vi "Measurement UI.vi"() -> ()   [LabVIEW 2024, in "Line Regulation_Channel Ganging_UI.lvlib"]
uses:
  Line Regulation_Channel Ganging_UI.lvlib
panel:
  in  "MeasGraphs":T1(tab)
  out "Enabled Sources":string[](array[string])
  out "Enabled Loads":string[](array[string])
  out "LineRegulationGraph(V/V)":T2(graph)
  out "LineRegulationGraph(%)":T3(graph)
  in  "Load current pole-zero ratio":dbl=0.3
  in  "Load current compensation frequency":dbl=180000.0
  in  "Load current gain bandwidth":dbl=14000.0
  in  "Source voltage pole-zero ratio":dbl=2.0
  in  "Source voltage compensation frequency":dbl=3530.0
  in  "Source voltage gain bandwidth":dbl=2000.0
  out "Load voltage deviation":dbl[](array[numeric])
  out "Ganged load voltages":dbl[](array[numeric])
  out "Ganged source voltages":dbl[](array[numeric])
  in  "Load slave resource names":string[](array[string])
  in  "Load master resource name":string
  in  "Source slave resource names":string[](array[string])
  in  "Source master resource name":string
  in  "Mode of operation":T4(ring)=enum."Perform measurement" caption="MODE OF OPERATION"
  in  "MeasConfigurations":T5(tab)=enum."Source Config"
  in  "Measurement timeout":dbl=10.0 caption="MEASUREMENT TIMEOUT" format="%.3ps"
  in  "Nominal output voltage":dbl=1.0 caption="NOMINAL OUTPUT VOLTAGE" format="%.3pV"
  in  "Source delay":dbl=0.005 caption="SOURCE DELAY" format="%.3ps"
  in  "DUT setup time":dbl=1.0 caption="DUT SETUP TIME" format="%.3ps"
  in  "Aperture time":dbl=0.005 caption="APERTURE TIME" format="%.3ps"
  in  "PPSSlaveResourceNames":refnum<k15>[](array[refnum]) caption="SLAVE RESOURCE NAMES"
  in  "PPSMasterResourceName":refnum<k15> caption="MASTER RESOURCE NAME"
  in  "Source stop voltage":dbl=14.0 caption="VOLTAGE STOP LEVEL" format="%#_6pV"
  in  "Source transient response":i32(ring)=1038 caption="TRANSIENT RESPONSE" items=["Slow"=1041, "Normal"=1038, "Fast"=1039, "Custom"=1042]
  in  "Source sense":i32(ring)=1009 caption="SENSE" items=["Local"=1008, "Remote"=1009]
  in  "Source voltage level range":dbl=20.0 caption="VOLTAGE LEVEL RANGE" format="%#_6pV"
  in  "Source start voltage":dbl=6.0 caption="VOLTAGE START LEVEL" format="%#_6pV"
  in  "Source current limit high":dbl=25.0 caption="CURRENT LIMIT/LIMIT HIGH" format="%#_6pA"
  in  "Source current limit range":dbl=25.0 caption="CURRENT LIMIT RANGE" format="%#_6pA"
  in  "Source limit symmetry":enum32{"Symmetric", "Asymmetric"}(ring)=enum."Asymmetric" caption="LIMIT SYMMETRY"
  in  "Source current limit low":dbl=-0.6 caption="CURRENT LIMIT LOW" format="%#_6pA"
  in  "Source system configuration":enum32{"Series", "Parallel"}(ring)=enum."Parallel" caption="SYSTEM CONFIG"
  in  "Source compliance":string="Compliance"
  in  "Source sourceadapt":string="SourceAdapt"
  in  "Source Custom Transient Response":bool
  in  "Source sweep type":string(combo)="Logarithmic" caption="SWEEP TYPE"
  in  "Source current sweep points/points per decade":i32=10 caption="PTS/PTS PER DECADE"
  out "Status":string
  in  "Load current level":dbl=1.0 caption="CURRENT LEVEL" format="%#_6pA"
  in  "Load sourceadapt":string="SourceAdapt"
  in  "Load compliance":string="Compliance"
  in  "Load system configuration":enum32{"Series", "Parallel"}(ring)=enum."Parallel" caption="SYSTEM CONFIG"
  in  "Load voltage limit low":dbl caption="VOLTAGE  LIMIT LOW" format="%#_6pV"
  in  "Load limit symmetry":enum32{"Symmetric", "Asymmetric"}(ring) caption="LIMIT SYMMETRY"
  in  "Load voltage limit range":dbl=6.0 caption="VOLTAGE LIMIT RANGE" format="%#_6pV"
  in  "Load voltage limit high":dbl=inf caption="VOLTAGE LIMIT/LIMIT HIGH" format="%#_6p"
  in  "Load current level range":dbl=80.0 caption="CURRENT LEVEL RANGE" format="%#_6pA"
  in  "Load sense":i32(ring)=1009 caption="SENSE" items=["Local"=1008, "Remote"=1009]
  in  "Load transient response":i32(ring)=1038 caption="TRANSIENT RESPONSE" items=["Slow"=1041, "Normal"=1038, "Fast"=1039, "Custom"=1042]
  in  "LoadSlaveResourceNames":refnum<k15>[](array[refnum]) caption="SLAVE RESOURCE NAMES"
  in  "LoadMasterResourceName":refnum<k15> caption="MASTER RESOURCE NAME"
  in  "Load Custom Transient Response":bool
  out "Status (Load)":string
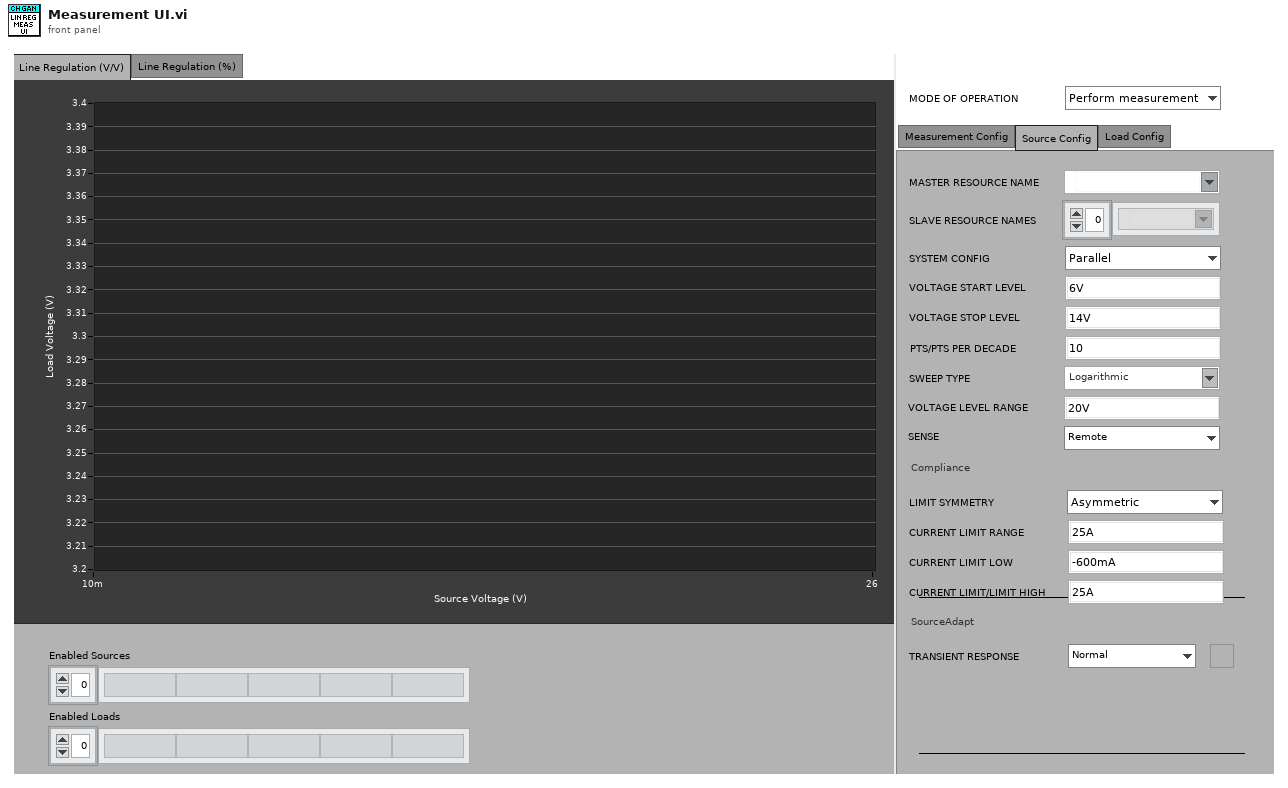
[diagram p1: front panel]
types:
  T1 = enum32{"Line Regulation (V/V)", "Line Regulation (%)", "Hidden Controls"}
  T2 = cluster{"Source voltages":dbl[], "Load voltages":dbl[]}
  T3 = cluster{"Source voltages":dbl[], "Load voltage deviation":dbl[]}
  T4 = enum32{"Power on the DUT", "Perform measurement", "Power off the DUT"}
  T5 = enum32{"Measurement Config", "Source Config", "Load Config"}
  T6 = typedef "SourceAdapt Parameters.ctl" = cluster{"Voltage gain bandwidth":dbl, "Voltage compensation frequency":dbl, "Voltage pole-zero ratio":dbl, "Current gain bandwidth":dbl, "Current compensation frequency":dbl, "Current pole-zero ratio":dbl}
  T7 = cluster{"Ganged source voltages":dbl[], "Ganged load voltages":dbl[]}
  T8 = cluster{"Ganged source voltages":dbl[], "Load voltage deviation":dbl[]}
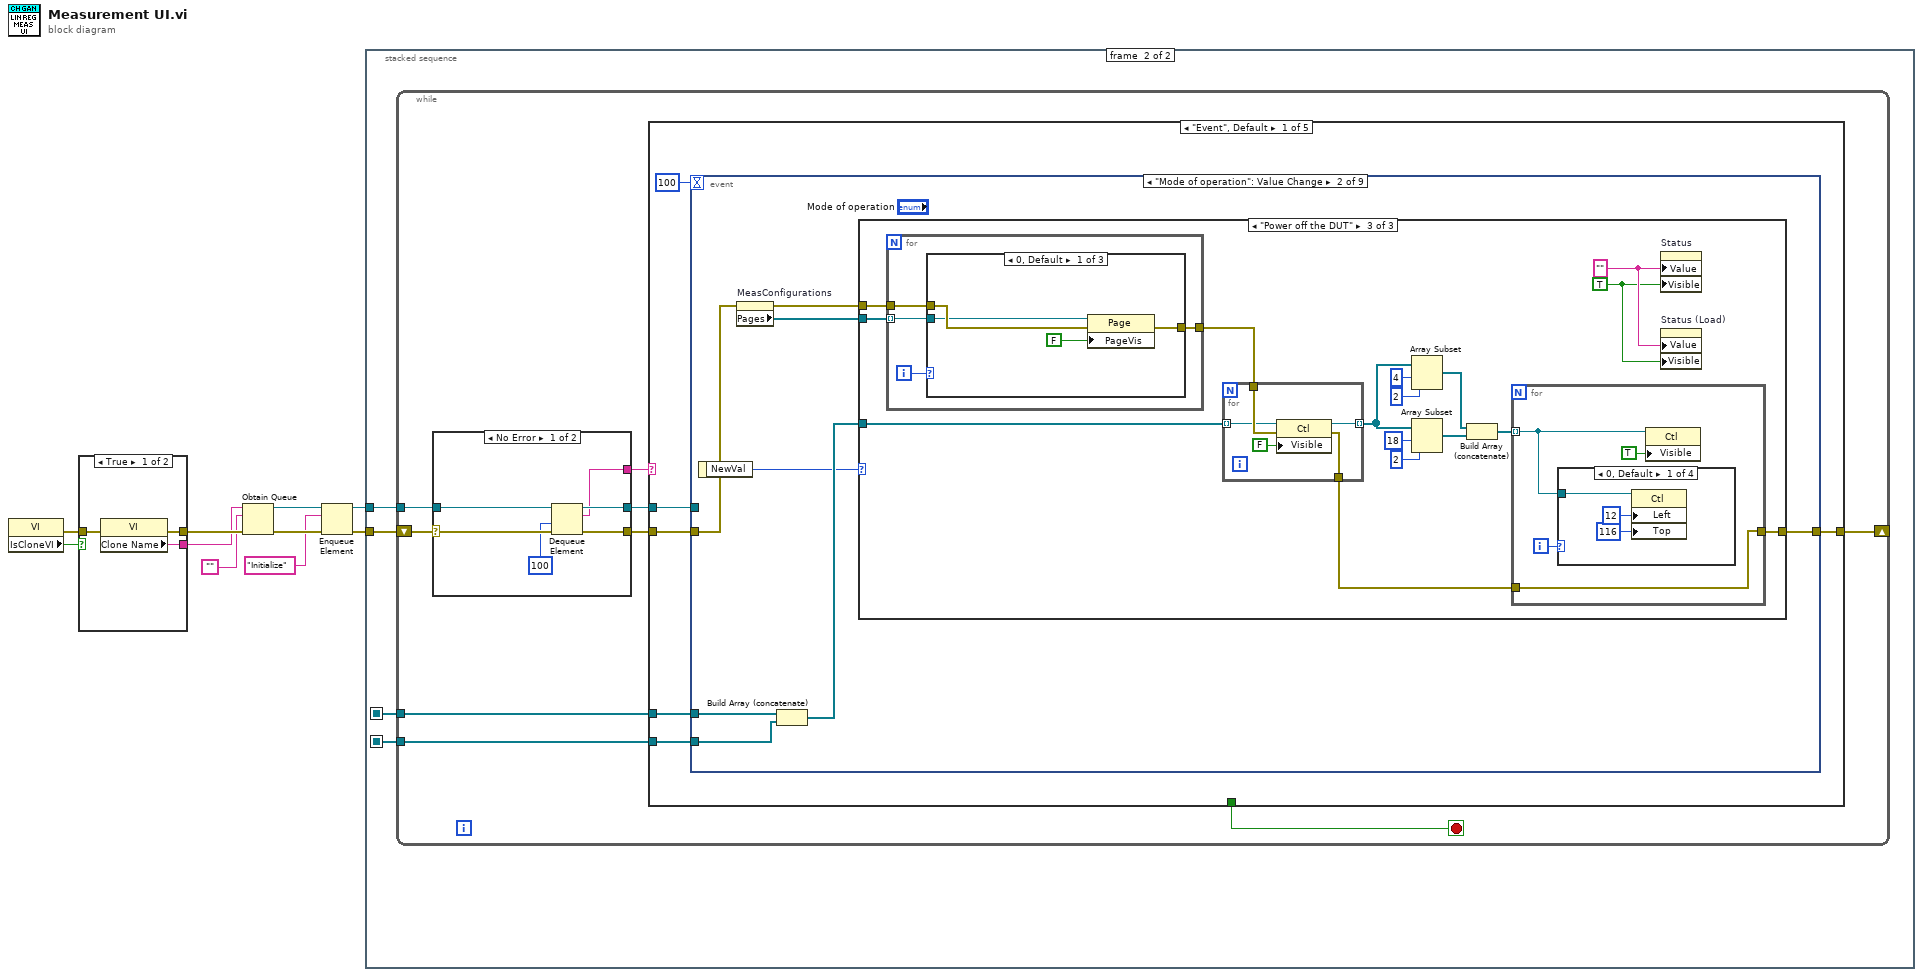
[diagram p0: block diagram]
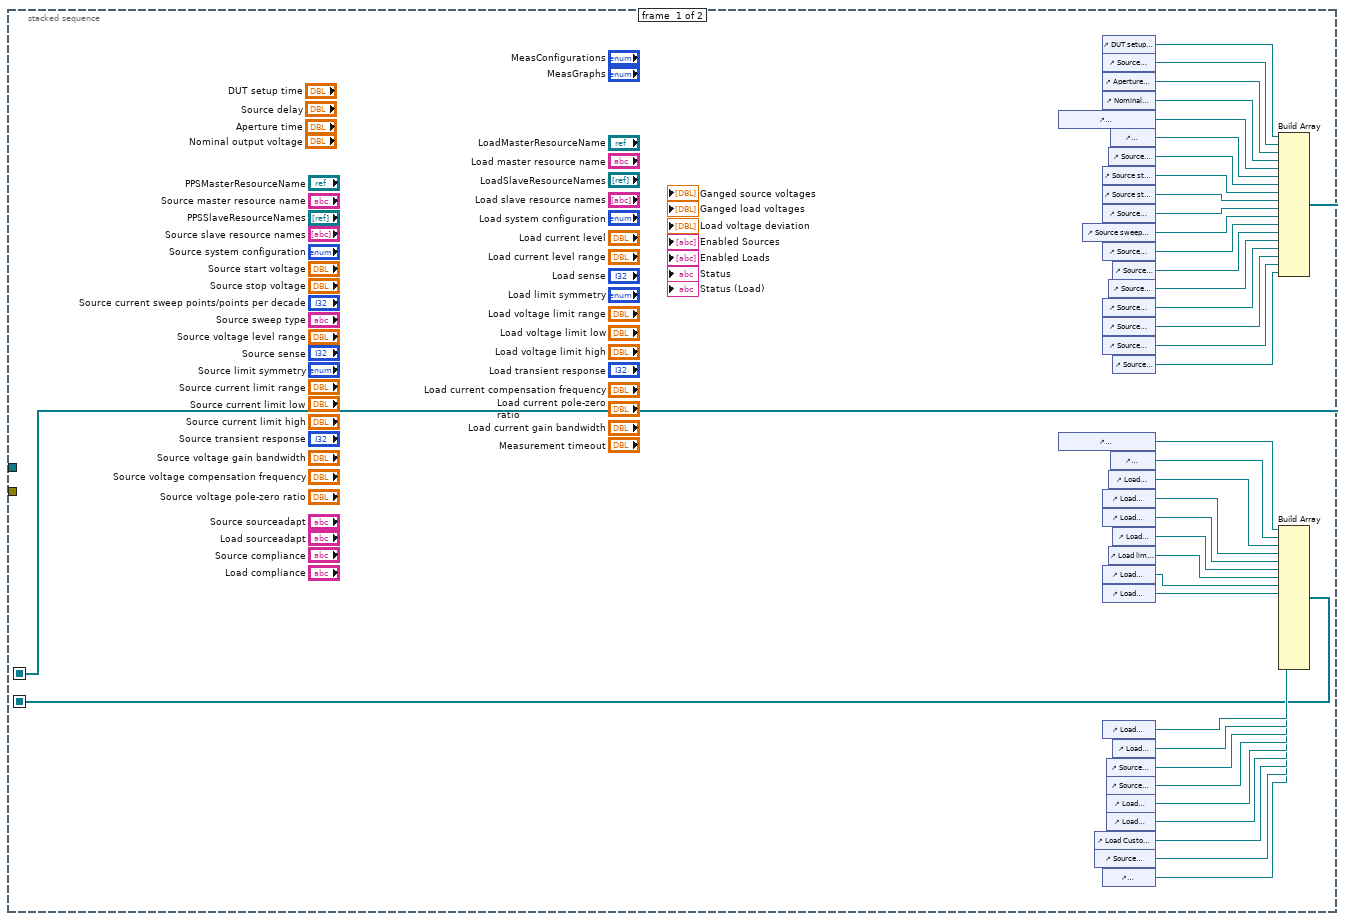
[diagram p2: hidden frame]
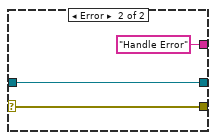
[diagram p3: hidden frame]
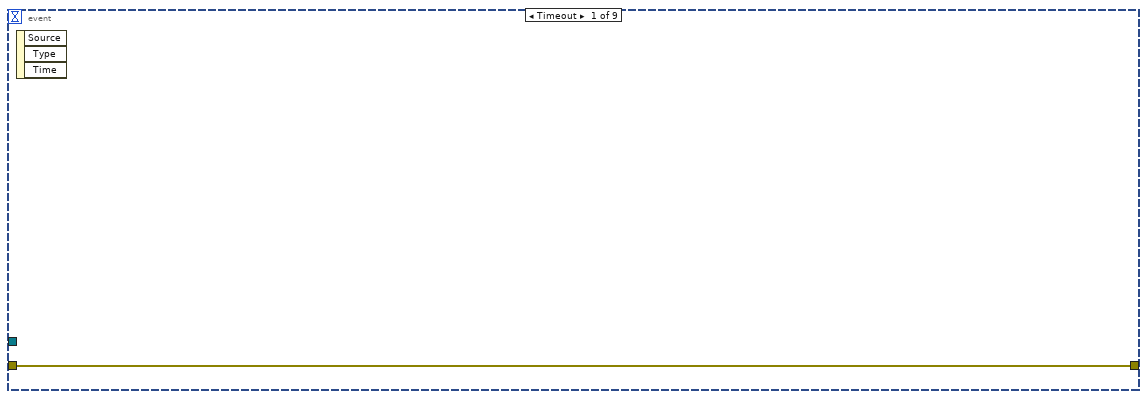
[diagram p4: hidden frame]
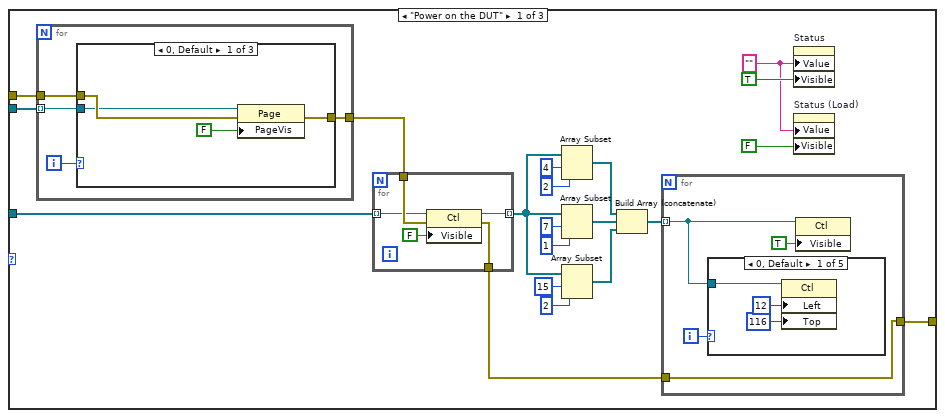
[diagram p5: hidden frame]
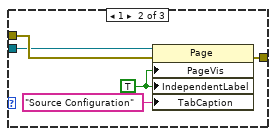
[diagram p6: hidden frame]
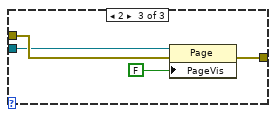
[diagram p7: hidden frame]
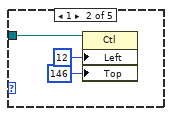
[diagram p8: hidden frame]
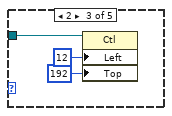
[diagram p9: hidden frame]
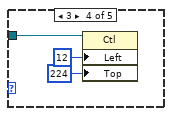
[diagram p10: hidden frame]
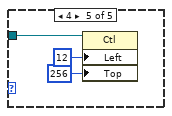
[diagram p11: hidden frame]
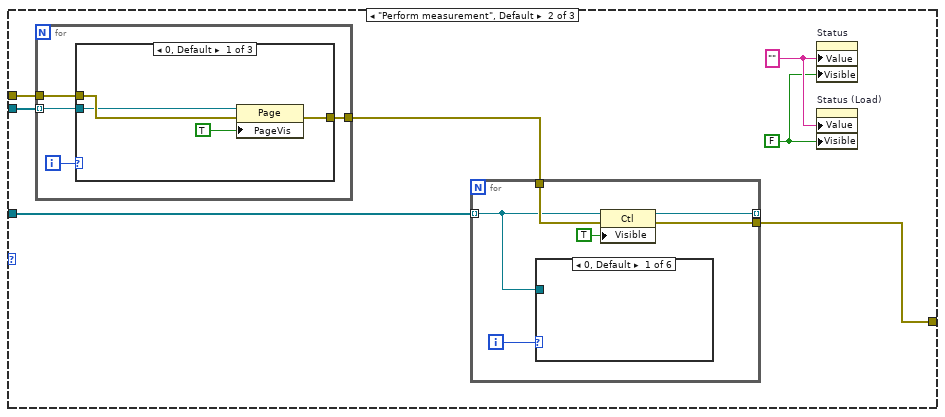
[diagram p12: hidden frame]
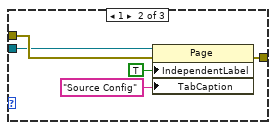
[diagram p13: hidden frame]
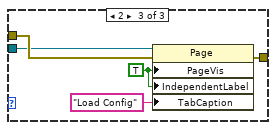
[diagram p14: hidden frame]
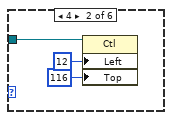
[diagram p15: hidden frame]
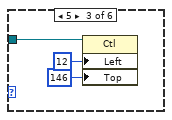
[diagram p16: hidden frame]
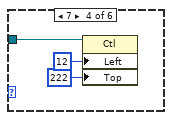
[diagram p17: hidden frame]
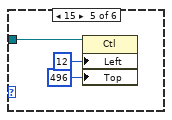
[diagram p18: hidden frame]
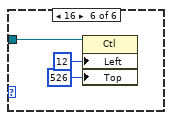
[diagram p19: hidden frame]
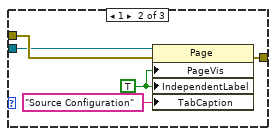
[diagram p20: hidden frame]
diagram:
  n1 = property class="VI"() -> (error out=w1:errorcluster, "IsCloneVI"=w2:bool)  [unwired: 2 in, 1 out]
  n2 = case shown="True" w2 {
    tunnel: [w13 w16] -> w10
    tunnel: [w12 w15] -> w9
    tunnel: w1 -> [w11 w14]
    frame True {
      n3 = property class="VI"(error in=w11) -> (error out=w13:errorcluster, "Clone Name"=w12:string)  [unwired: 1 in, 1 out]
    }
    frame False {
      n4 = property class="VI"(error in=w14) -> (error out=w16:errorcluster, "Name"=w15:string)  [unwired: 1 in, 1 out]
    }
  }
  n5 = Obtain Queue(name (unnamed)=w9, element data type="", error in (no error)=w10) -> (queue out=w6:refnum<queue>, error out=w8:errorcluster)  [unwired: 2 in, 1 out]
  n6 = Enqueue Element(queue=w6, element="Initialize", error in (no error)=w8) -> (queue out=w5:refnum<queue>, error out=w7:errorcluster)  [unwired: 1 in, 1 out]
  n7 = stacked-sequence {
    seq-local: [w18 _] -> [_ w56]
    seq-local: [w17 _] -> [_ w55]
    tunnel: w7 -> [_ w58]
    tunnel: w5 -> [_ w57]
    frame #0 {
      n8 = control-ref of="PPSMasterResourceName"() -> (w50:refnum<vi>)
      n9 = control-ref of="LoadMasterResourceName"() -> (w36:refnum<vi>)
      n10 = control-ref of="Source sweep type"() -> (w44:refnum<vi>)
      n11 = control-ref of="Load Custom Transient Response"() -> (w21:refnum<vi>)
      n12 = control-ref of="Source Custom Transient Response"() -> (w20:refnum<vi>)
      n13 = control-ref of="DUT setup time"() -> (w54:refnum<vi>)
      n14 = control-ref of="Source delay"() -> (w53:refnum<vi>)
      n15 = control-ref of="Aperture time"() -> (w52:refnum<vi>)
      n16 = control-ref of="Nominal output voltage"() -> (w51:refnum<vi>)
      n17 = control-ref of="Source start voltage"() -> (w47:refnum<vi>)
      n18 = control-ref of="Source stop voltage"() -> (w46:refnum<vi>)
      n19 = control-ref of="Source current sweep points/points per decade"() -> (w45:refnum<vi>)
      n20 = control-ref of="Source voltage level range"() -> (w43:refnum<vi>)
      n21 = control-ref of="Source current limit range"() -> (w40:refnum<vi>)
      n22 = control-ref of="Source current limit low"() -> (w39:refnum<vi>)
      n23 = control-ref of="Source current limit high"() -> (w38:refnum<vi>)
      n24 = control-ref of="Load current level"() -> (w33:refnum<vi>)
      n25 = control-ref of="Load current level range"() -> (w32:refnum<vi>)
      n26 = control-ref of="Load voltage limit range"() -> (w29:refnum<vi>)
      n27 = control-ref of="Load voltage limit low"() -> (w28:refnum<vi>)
      n28 = control-ref of="Load voltage limit high"() -> (w27:refnum<vi>)
      n29 = control-ref of="Measurement timeout"() -> (w19:refnum<vi>)
      n30 = control-ref of="Source compliance"() -> (w25:refnum<vi>)
      n31 = control-ref of="Source sourceadapt"() -> (w24:refnum<vi>)
      n32 = control-ref of="Load compliance"() -> (w23:refnum<vi>)
      n33 = control-ref of="Load sourceadapt"() -> (w22:refnum<vi>)
      n34 = control-ref of="Source system configuration"() -> (w48:refnum<vi>)
      n35 = control-ref of="Source limit symmetry"() -> (w41:refnum<vi>)
      n36 = control-ref of="Load system configuration"() -> (w34:refnum<vi>)
      n37 = control-ref of="Load limit symmetry"() -> (w30:refnum<vi>)
      n38 = control-ref of="PPSSlaveResourceNames"() -> (w49:refnum<vi>)
      n39 = control-ref of="LoadSlaveResourceNames"() -> (w35:refnum<vi>)
      n40 = control-ref of="Source sense"() -> (w42:refnum<vi>)
      n41 = control-ref of="Source transient response"() -> (w37:refnum<vi>)
      n42 = control-ref of="Load sense"() -> (w31:refnum<vi>)
      n43 = control-ref of="Load transient response"() -> (w26:refnum<vi>)
      n44 = Build Array(w54, w53, w52, w51, w50, w49, w48, w47, w46, w45, w44, w43, w42, w41, w40, w39, w38, w37) -> (w18:refnum<vi>[])
      n45 = Build Array(w36, w35, w34, w33, w32, w31, w30, w29, w28, w27, w26, w25, w24, w23, w22, w21, w20, w19) -> (w17:refnum<vi>[])
    }
    frame #1 {
      n46 = while {
        shift-right: [w62] -> _
        shift-left: w58 -> [w67]
        tunnel: w57 -> [w65]
        tunnel: w56 -> [w60]
        tunnel: w55 -> [w59]
        stop <- w61 stop-if-true
        n47 = case shown="No Error" w67 {
          selector: w67 -> [w73 w76]
          tunnel: [w72 w76] -> w66
          tunnel: w65 -> [w71 w75]
          tunnel: [w70 w75] -> w64
          tunnel: [w69 "Handle Error"] -> w63
          frame No Error {
            n48 = Dequeue Element(queue=w71, timeout in ms (-1)=100, error in (no error)=w73) -> (queue out=w70:refnum<queue>, element=w69:string, error out=w72:errorcluster)  [unwired: 1 out]
          }
          frame Error {
          }
        }
        n49 = case shown="\"Event\", Default" w63 {
          tunnel: w66 -> [w81 w272 w285 w294 w295]
          tunnel: w64 -> [w79 _ _ w292 _]
          tunnel: [w82 w272 w285 w289 w295] -> w62
          tunnel: [_ FALSE _ TRUE _] -> w61
          tunnel: w60 -> [w78 _ _ _ _]
          tunnel: w59 -> [w77 _ _ _ _]
          frame "Event", Default {
            n50 = event shown="[1] \"Mode of operation\": Value Change" {
              selector: _ -> [_ _ _ _ _ _ _ _ _]
              dyn-events: _ -> [_ _ _ _ _ _ _ _ _]
              timeout: 100 -> [_ _ _ _ _ _ _ _ _]
              tunnel: [w83 w90 _ _ _ _ _ _ w268] -> w82
              tunnel: w81 -> [w83 w84 _ _ _ _ _ _ w269]
              tunnel: w79 -> [_ _ _ _ _ _ _ _ w267]
              tunnel: w78 -> [_ w88 _ _ _ _ _ _ _]
              tunnel: w77 -> [_ w87 _ _ _ _ _ _ _]
              event Timeout {
                n51 = event-data() -> ()  [unwired: 1 in, 3 out]
              }
              event "Mode of operation": Value Change {
                n52 = event-data() -> ("NewVal"=w89:T4)  [unwired: 1 in]
                n53 = property on="MeasConfigurations" class="TabCtl (strict)"(error in=w84) -> (error out=w85:errorcluster, "Pages"=w86:refnum<vi>[])  [unwired: 1 in, 1 out]
                n54 = Build Array (concatenate)(w88, w87) -> (w91:refnum<vi>[])
                n55 = case shown="\"Power off the DUT\"" w89 {
                  tunnel: w91 -> [w111 w159 w214]
                  tunnel: w86 -> [w99 w158 w209]
                  tunnel: w85 -> [w98 w157 w208]
                  tunnel: [w95 w155 w205] -> w90
                  frame "Power on the DUT" {
                    w93 = ""
                    n56 = for {
                      tunnel: w99 -> [w114] mode=indexing
                      tunnel: w98 -> [w113]
                      tunnel: [w112] -> w97
                      i -> [w115]
                      n57 = case shown="0, Default" w115 {
                        tunnel: w114 -> [w118 w123 w127]
                        tunnel: w113 -> [w119 w124 w128]
                        tunnel: [w116 w121 w125] -> w112
                        frame 0, Default {
                          n58 = property class="Page"(reference=w118, error in=w119, "PageVis"=FALSE ("Independent Label")) -> (error out=w116:errorcluster)  [unwired: 1 out]
                        }
                        frame 1 {
                          w120 = TRUE ("Independent Label")
                          n59 = property class="Page"(reference=w123, error in=w124, "PageVis"=w120, "IndependentLabel"=w120, "TabCaption"="Source Configuration" ("Tab Caption")) -> (error out=w121:errorcluster)  [unwired: 1 out]
                        }
                        frame 2 {
                          n60 = property class="Page"(reference=w127, error in=w128, "PageVis"=FALSE ("Independent Label")) -> (error out=w125:errorcluster)  [unwired: 1 out]
                        }
                      }
                    }
                    n61 = for {
                      tunnel: w111 -> [w151] mode=indexing
                      tunnel: [w149] -> w104 mode=indexing
                      tunnel: w97 -> [w152]
                      tunnel: [w148] -> w96
                      n62 = property class="Ctl"(reference=w151, error in=w152, "Visible"=FALSE) -> (reference out=w149:refnum<vi>, error out=w148:errorcluster)
                    }
                    n63 = Array Subset(array=w104, index=4, length=2) -> (w102:refnum<vi>[])
                    n64 = Array Subset(array=w104, index=7, length=1) -> (w103:refnum<vi>[])
                    n65 = Array Subset(array=w104, index=15, length=2) -> (w101:refnum<vi>[])
                    n66 = Build Array (concatenate)(w102, w103, w101) -> (w100:refnum<vi>[])
                    n67 = for {
                      tunnel: w100 -> [w130] mode=indexing
                      tunnel: w96 -> [w129]
                      tunnel: [w129] -> w95
                      i -> [w131]
                      n68 = case shown="0, Default" w131 {
                        tunnel: w130 -> [w135 w138 w141 w144 w147]
                        frame 0, Default {
                          n69 = property class="Ctl"(reference=w135, "Left"=12 ("Position:Left"), "Top"=116 ("Position:Left")) -> ()  [unwired: 1 in, 2 out]
                        }
                        frame 1 {
                          n70 = property class="Ctl"(reference=w138, "Left"=12 ("Position:Left"), "Top"=146 ("Position:Left")) -> ()  [unwired: 1 in, 2 out]
                        }
                        frame 2 {
                          n71 = property class="Ctl"(reference=w141, "Left"=12 ("Position:Left"), "Top"=192 ("Position:Left")) -> ()  [unwired: 1 in, 2 out]
                        }
                        frame 3 {
                          n72 = property class="Ctl"(reference=w144, "Left"=12 ("Position:Left"), "Top"=224 ("Position:Left")) -> ()  [unwired: 1 in, 2 out]
                        }
                        frame 4 {
                          n73 = property class="Ctl"(reference=w147, "Left"=12 ("Position:Left"), "Top"=256 ("Position:Left")) -> ()  [unwired: 1 in, 2 out]
                        }
                      }
                      n74 = property class="Ctl"(reference=w130, "Visible"=TRUE) -> ()  [unwired: 1 in, 2 out]
                    }
                    n75 = property on="Status" class="Str"("Value"=w93, "Visible"=TRUE) -> ()  [unwired: 2 in, 2 out]
                    n76 = property on="Status (Load)" class="Str"("Value"=w93, "Visible"=FALSE) -> ()  [unwired: 2 in, 2 out]
                  }
                  frame "Perform measurement", Default {
                    w153 = FALSE ("Visible")
                    w154 = ""
                    n77 = for {
                      tunnel: w158 -> [w162] mode=indexing
                      tunnel: w157 -> [w161]
                      tunnel: [w160] -> w156
                      i -> [w163]
                      n78 = case shown="0, Default" w163 {
                        tunnel: w162 -> [w166 w171 w176]
                        tunnel: w161 -> [w167 w172 w177]
                        tunnel: [w164 w168 w175] -> w160
                        frame 0, Default {
                          n79 = property class="Page"(reference=w166, error in=w167, "PageVis"=TRUE ("Independent Label")) -> (error out=w164:errorcluster)  [unwired: 1 out]
                        }
                        frame 1 {
                          n80 = property class="Page"(reference=w171, error in=w172, "IndependentLabel"=TRUE ("Independent Label"), "TabCaption"="Source Config" ("Tab Caption")) -> (error out=w168:errorcluster)  [unwired: 1 out]
                        }
                        frame 2 {
                          w174 = TRUE ("Independent Label")
                          n81 = property class="Page"(reference=w176, error in=w177, "PageVis"=w174, "IndependentLabel"=w174, "TabCaption"="Load Config" ("Tab Caption")) -> (error out=w175:errorcluster)  [unwired: 1 out]
                        }
                      }
                    }
                    n82 = for {
                      tunnel: w159 -> [w179] mode=indexing
                      tunnel: [w181] -> _ mode=indexing
                      tunnel: w156 -> [w183]
                      tunnel: [w178] -> w155
                      i -> [w180]
                      n83 = case shown="0, Default" w180 {
                        tunnel: w179 -> [_ w186 w189 w192 w195 w198]
                        frame 0, Default {
                        }
                        frame 4 {
                          n84 = property class="Ctl"(reference=w186, "Left"=12 ("Position:Left"), "Top"=116 ("Position:Left")) -> ()  [unwired: 1 in, 2 out]
                        }
                        frame 5 {
                          n85 = property class="Ctl"(reference=w189, "Left"=12 ("Position:Left"), "Top"=146 ("Position:Left")) -> ()  [unwired: 1 in, 2 out]
                        }
                        frame 7 {
                          n86 = property class="Ctl"(reference=w192, "Left"=12 ("Position:Left"), "Top"=222 ("Position:Left")) -> ()  [unwired: 1 in, 2 out]
                        }
                        frame 15 {
                          n87 = property class="Ctl"(reference=w195, "Left"=12 ("Position:Left"), "Top"=496 ("Position:Left")) -> ()  [unwired: 1 in, 2 out]
                        }
                        frame 16 {
                          n88 = property class="Ctl"(reference=w198, "Left"=12 ("Position:Left"), "Top"=526 ("Position:Left")) -> ()  [unwired: 1 in, 2 out]
                        }
                      }
                      n89 = property class="Ctl"(reference=w179, error in=w183, "Visible"=TRUE) -> (reference out=w181:refnum<vi>, error out=w178:errorcluster)
                    }
                    n90 = property on="Status" class="Str"("Value"=w154, "Visible"=w153) -> ()  [unwired: 2 in, 2 out]
                    n91 = property on="Status (Load)" class="Str"("Value"=w154, "Visible"=w153) -> ()  [unwired: 2 in, 2 out]
                  }
                  frame "Power off the DUT" {
                    w199 = TRUE
                    w200 = ""
                    n92 = for {
                      tunnel: w209 -> [w217] mode=indexing
                      tunnel: w208 -> [w216]
                      tunnel: [w215] -> w207
                      i -> [w218]
                      n93 = case shown="0, Default" w218 {
                        tunnel: w217 -> [w221 w226 w231]
                        tunnel: w216 -> [w222 w227 w232]
                        tunnel: [w219 w224 w229] -> w215
                        frame 0, Default {
                          n94 = property class="Page"(reference=w221, error in=w222, "PageVis"=FALSE ("Independent Label")) -> (error out=w219:errorcluster)  [unwired: 1 out]
                        }
                        frame 1 {
                          w223 = TRUE ("Independent Label")
                          n95 = property class="Page"(reference=w226, error in=w227, "PageVis"=w223, "IndependentLabel"=w223, "TabCaption"="Source Configuration" ("Tab Caption")) -> (error out=w224:errorcluster)  [unwired: 1 out]
                        }
                        frame 2 {
                          w228 = TRUE ("Independent Label")
                          n96 = property class="Page"(reference=w231, error in=w232, "PageVis"=w228, "IndependentLabel"=w228, "TabCaption"="Load Configuration" ("Tab Caption")) -> (error out=w229:errorcluster)  [unwired: 1 out]
                        }
                      }
                    }
                    n97 = for {
                      tunnel: w214 -> [w252] mode=indexing
                      tunnel: [w250] -> w202 mode=indexing
                      tunnel: w207 -> [w253]
                      tunnel: [w249] -> w206
                      n98 = property class="Ctl"(reference=w252, error in=w253, "Visible"=FALSE) -> (reference out=w250:refnum<vi>, error out=w249:errorcluster)
                    }
                    n99 = Array Subset(array=w202, index=4, length=2) -> (w211:refnum<vi>[])
                    n100 = Array Subset(array=w202, index=18, length=2) -> (w201:refnum<vi>[])
                    n101 = Build Array (concatenate)(w211, w201) -> (w210:refnum<vi>[])
                    n102 = for {
                      tunnel: w210 -> [w234] mode=indexing
                      tunnel: w206 -> [w233]
                      tunnel: [w233] -> w205
                      i -> [w235]
                      n103 = case shown="0, Default" w235 {
                        tunnel: w234 -> [w239 w242 w245 w248]
                        frame 0, Default {
                          n104 = property class="Ctl"(reference=w239, "Left"=12 ("Position:Left"), "Top"=116 ("Position:Left")) -> ()  [unwired: 1 in, 2 out]
                        }
                        frame 1 {
                          n105 = property class="Ctl"(reference=w242, "Left"=12 ("Position:Left"), "Top"=146 ("Position:Left")) -> ()  [unwired: 1 in, 2 out]
                        }
                        frame 2 {
                          n106 = property class="Ctl"(reference=w245, "Left"=12 ("Position:Left"), "Top"=116 ("Position:Left")) -> ()  [unwired: 1 in, 2 out]
                        }
                        frame 3 {
                          n107 = property class="Ctl"(reference=w248, "Left"=12 ("Position:Left"), "Top"=146 ("Position:Left")) -> ()  [unwired: 1 in, 2 out]
                        }
                      }
                      n108 = property class="Ctl"(reference=w234, "Visible"=TRUE) -> ()  [unwired: 1 in, 2 out]
                    }
                    n109 = property on="Status" class="Str"("Value"=w200, "Visible"=w199) -> ()  [unwired: 2 in, 2 out]
                    n110 = property on="Status (Load)" class="Str"("Value"=w200, "Visible"=w199) -> ()  [unwired: 2 in, 2 out]
                  }
                }
              }
              event "PPSMasterResourceName": Value Change {
                n111 = event-data() -> ("NewVal"=w254:refnum<k15>)  [unwired: 1 in]
                n112 = property on="Source master resource name" class="Str"("Value"=w254) -> ()  [unwired: 2 in, 2 out]
              }
              event "PPSSlaveResourceNames": Value Change {
                n113 = event-data() -> ("NewVal"=w255:refnum<k15>[])  [unwired: 1 in]
                n114 = property on="Source slave resource names" class="Arr (strict)"("Value"=w255) -> ()  [unwired: 2 in, 2 out]
              }
              event "LoadMasterResourceName": Value Change {
                n115 = event-data() -> ("NewVal"=w256:refnum<k15>)  [unwired: 1 in]
                n116 = property on="Load master resource name" class="Str"("Value"=w256) -> ()  [unwired: 2 in, 2 out]
              }
              event "LoadSlaveResourceNames": Value Change {
                n117 = event-data() -> ("NewVal"=w257:refnum<k15>[])  [unwired: 1 in]
                n118 = property on="Load slave resource names" class="Arr (strict)"("Value"=w257) -> ()  [unwired: 2 in, 2 out]
              }
              event "Source Custom Transient Response": Value Change {
                n119 = event-data() -> ()  [unwired: 1 in, 6 out]
                n120 = call "Custom Transient Response for Sweep & Single Point.vi"() -> ("SourceAdapt Parameters"=w261:T6)  [unwired: 11 in]
                n121 = Unbundle By Name(w261) -> ("Voltage gain bandwidth"=w260:dbl, "Voltage compensation frequency"=w259:dbl, "Voltage pole-zero ratio"=w258:dbl)
                n122 = property on="Source voltage gain bandwidth" class="DigNum (strict)"("Value"=w260) -> ()  [unwired: 2 in, 2 out]
                n123 = property on="Source voltage compensation frequency" class="DigNum (strict)"("Value"=w259) -> ()  [unwired: 2 in, 2 out]
                n124 = property on="Source voltage pole-zero ratio" class="DigNum (strict)"("Value"=w258) -> ()  [unwired: 2 in, 2 out]
              }
              event "Load Custom Transient Response": Value Change {
                n125 = event-data() -> ()  [unwired: 1 in, 6 out]
                n126 = call "Custom Transient Response for Sweep & Single Point.vi"() -> ("SourceAdapt Parameters"=w265:T6)  [unwired: 11 in]
                n127 = Unbundle By Name(w265) -> ("Current gain bandwidth"=w264:dbl, "Current compensation frequency"=w263:dbl, "Current pole-zero ratio"=w262:dbl)
                n128 = property on="Load current gain bandwidth" class="DigNum (strict)"("Value"=w264) -> ()  [unwired: 2 in, 2 out]
                n129 = property on="Load current compensation frequency" class="DigNum (strict)"("Value"=w263) -> ()  [unwired: 2 in, 2 out]
                n130 = property on="Load current pole-zero ratio" class="DigNum (strict)"("Value"=w262) -> ()  [unwired: 2 in, 2 out]
              }
              event Panel Close? {
                n131 = event-data() -> ()  [unwired: 1 in, 4 out]
                n132 = Enqueue Element(queue=w267, element="Exit", error in (no error)=w269) -> (error out=w268:errorcluster)  [unwired: 1 in, 2 out]
                n133 = event-data("Discard?"=TRUE) -> ()  [unwired: 1 in, 1 out]
              }
            }
          }
          frame "Initialize" {
          }
          frame "Post UI Update" {
            # "This case will be triggered, after framework updates the User interface with result values."
            n134 = local read "Source sweep type"() -> (w280:string)
            n135 = control-ref of="LineRegulationGraph(%)"() -> (w278:refnum<vi>)
            n136 = control-ref of="LineRegulationGraph(V/V)"() -> (w279:refnum<vi>)
            n137 = local read "Ganged source voltages"() -> (w275:dbl[])
            n138 = local read "Ganged load voltages"() -> (w276:dbl[])
            n139 = local read "Load voltage deviation"() -> (w274:dbl[])
            n140 = Not Equal?(x="Linear", y=w280) -> (x != y?=w284:bool)
            n141 = Build Array(w279, w278) -> (w282:refnum<vi>[])
            n142 = Boolean To (0,1)(Boolean=w284) -> (0, 1=w283:i16)
            n143 = for {
              tunnel: w282 -> [w287] mode=indexing
              tunnel: w283 -> [w286]
              n144 = property class="XYGraph (strict)"(reference=w287, "XScale.Mapping Mode"=w286) -> ()  [unwired: 1 in, 2 out]
            }
            n145 = Bundle("Ganged source voltages"=w275, "Ganged load voltages"=w276) -> (→"LineRegulationGraph(V/V)":T7)  [unwired: 1 in]
            n146 = Bundle("Ganged source voltages"=w275, "Load voltage deviation"=w274) -> (→"LineRegulationGraph(%)":T8)  [unwired: 1 in]
          }
          frame "Exit" {
            # "This case is triggered to close the User Interface from framework"
            n147 = Flush Queue(queue=w292, error in (no error)=w294) -> (queue out=w291:refnum<queue>, error out=w290:errorcluster)  [unwired: 1 out]
            n148 = Release Queue(queue=w291, force destroy? (F)=TRUE, error in (no error)=w290) -> (error out=w289:errorcluster)  [unwired: 2 out]
          }
          frame "Handle Error" {
          }
        }
      }
    }
  }
